vi "Open file in hex view.vi"(8 "error in":errorcluster, 11 "file path":path) -> (0 "error out":errorcluster, 3 "hex display":string)   [LabVIEW 2016]
doc: "Open file from <b>file path</b> and return the <b>hex display</b> of its content."
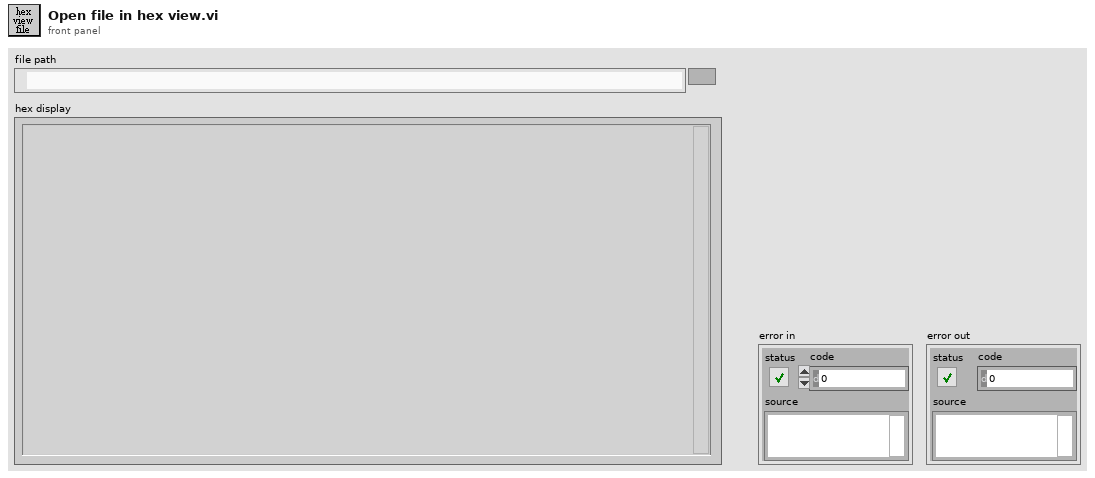
[diagram p1: front panel]
types:
  T1 = enum16{"open", "replace", "create", "open or create", "replace or create", "replace or create with confirmation"}
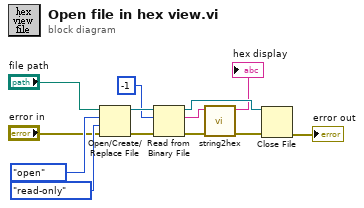
[diagram p0: block diagram]
diagram:
  n1 = Open/Create/Replace File(file path (use dialog)="file path", error in="error in", operation (0:open)=T1."open", access (0:read/write)=enum16{"read/write", "read-only", "write-only"}."read-only") -> (refnum out=w10:refnum<file>, error out=w9:errorcluster)  [unwired: 2 in, 1 out]
  n2 = Read from Binary File(8:w9, 10:-1 ("count (1)"), 11:w10) -> (0:w8:errorcluster, 2:w5:string, 3:w6:refnum<file>)  [unwired: 3 in, 1 out]
  n3 = call "string2hex.vi"("error in (no error)"=w8, "data input"=w5) -> ("error out"=w7:errorcluster, "hex display"=→"hex display":string)  [unwired: 8 in]
  n4 = Close File(refnum=w6, error in=w7) -> (error out=→"error out":errorcluster)  [unwired: 1 out]
